vi "niFpgaPID_PIDCore.vi"(0 "setpoint":sgl, 1 "reset? (F)":bool, 3 "channel (0)":u8, 5 "process variable":sgl, 7 "manual control":T2, 12 "gains":T5 {"filter coefficient" min=0 max=1; "proportional gain" step=0.125}, 13 "output range":T4={"output high (Inf)"=inf, "output low (-Inf)"=-inf}, 14 "setpoint weighting":T3={"proportional weighting (1)"=1.0, "derivative weighting (0)"=0.0} {"derivative weighting (0)" min=0 max=1; "proportional weighting (1)" min=0 max=1}) -> (4 "output":sgl, 6 "error":sgl, 8 "actions":T1)   [LabVIEW 2017]
uses:
  <vilib>/rvi/Analysis/control/PID/Typedef/niFpgaPID_PIDGains.ctl
  <vilib>/rvi/Analysis/control/PID/Typedef/niFpgaPID_OutputRange.ctl
  <vilib>/rvi/Analysis/control/PID/Typedef/niFpgaPID_SetpointWeightings.ctl
  <vilib>/rvi/Analysis/control/PID/Typedef/niFpgaPID_ManualControl.ctl
  <vilib>/rvi/Analysis/control/PID/Typedef/niFpgaPID_PIDActions.ctl
  <vilib>/rvi/Analysis/control/PID/Typedef/niFpgaPID_PIDParameters.ctl
  <vilib>/rvi/Analysis/control/PID/Typedef/niFpgaPID_PIDErrors.ctl
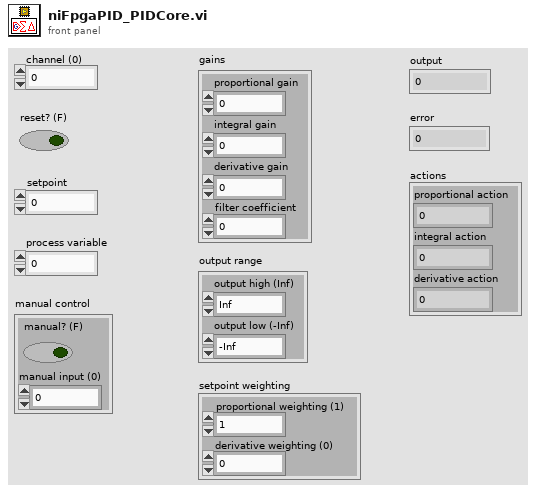
[diagram p1: front panel]
types:
  T1 = typedef "niFpgaPID_PIDActions.ctl" = cluster{"proportional action":sgl, "integral action":sgl, "derivative action":sgl}
  T2 = typedef "niFpgaPID_ManualControl.ctl" = cluster{"manual? (F)":bool, "manual input (0)":sgl}
  T3 = typedef "niFpgaPID_SetpointWeightings.ctl" = cluster{"proportional weighting (1)":sgl, "derivative weighting (0)":sgl}
  T4 = typedef "niFpgaPID_OutputRange.ctl" = cluster{"output high (Inf)":sgl, "output low (-Inf)":sgl}
  T5 = typedef "niFpgaPID_PIDGains.ctl" = cluster{"proportional gain":sgl, "integral gain":sgl, "derivative gain":sgl, "filter coefficient":sgl}
  T6 = typedef "niFpgaPID_PIDErrors.ctl" = cluster{"error":sgl, "error with beta":sgl, "error with gamma":sgl}
  T7 = typedef "niFpgaPID_PIDParameters.ctl" = cluster{"Kp":sgl, "Ki":sgl, "Kd":sgl, "manual?":bool, "beta":sgl}
  T8 = typedef "niFpgaPID_PIDState.ctl" = cluster{"uI(k-1)":sgl, "e(k-1)":sgl, "e(k-1) with gamma":sgl, "output (k-1)":sgl, "uD(k-1)":sgl}
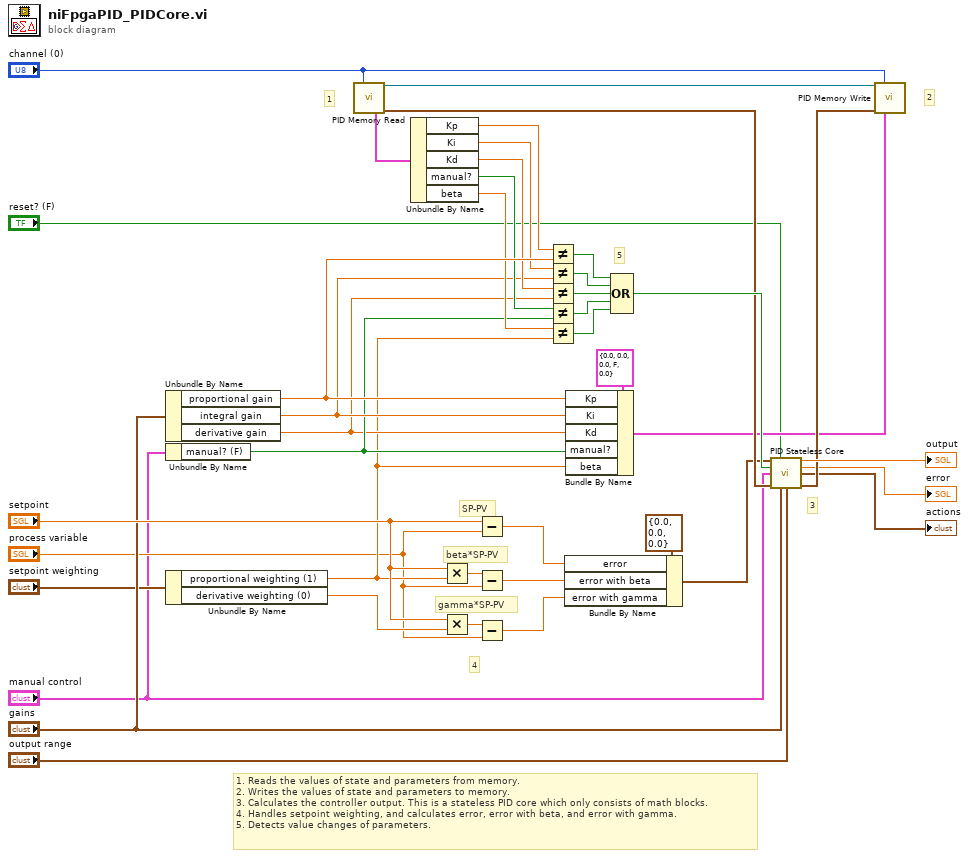
[diagram p0: block diagram]
diagram:
  # "SP-PV"
  # "beta*SP-PV"
  # "gamma*SP-PV"
  # "1. Reads the values of state and parameters from memory.\n2. Writes the values of state and parameters to memory.\n3. Calculates the controller output. This is a stateless PID core which only consists of math blocks.\n4. Handles setpoint weighting, and calculates error, error with beta, and error with gamma.\n5. Detects value changes of parameters."
  # "5"
  # "4"
  # "3"
  # "2"
  # "1"
  n1 = Unbundle By Name("gains") -> ("proportional gain"=w37:sgl, "integral gain"=w29:sgl, "derivative gain"=w27:sgl)
  n2 = Unbundle By Name("manual control") -> ("manual? (F)"=w28:bool)
  n3 = Unbundle By Name("setpoint weighting") -> ("proportional weighting (1)"=w16:sgl, "derivative weighting (0)"=w39:sgl)
  n4 = call "PID Memory Read"("channel (0)"="channel (0)") -> ("memory out"=w14:refnum<k21>, "parameters out"=w13:T7, "state out"=w35:T8)  [unwired: 12 in]
  n5 = Unbundle By Name(w13) -> ("Kp"=w34:sgl, "Ki"=w33:sgl, "Kd"=w32:sgl, "manual?"=w31:bool, "beta"=w30:sgl)
  n6 = Multiply(x="setpoint", y=w16) -> (x*y=w1:sgl)
  n7 = Multiply(x="setpoint", y=w39) -> (x*y=w2:sgl)
  n8 = Subtract(x="setpoint", y="process variable") -> (x-y=w5:sgl)
  n9 = Subtract(x=w1, y="process variable") -> (x-y=w10:sgl)
  n10 = Subtract(x=w2, y="process variable") -> (x-y=w9:sgl)
  n11 = Not Equal?(x=w34, y=w37) -> (x != y?=w26:bool)
  n12 = Not Equal?(x=w33, y=w29) -> (x != y?=w25:bool)
  n13 = Not Equal?(x=w32, y=w27) -> (x != y?=w24:bool)
  n14 = Not Equal?(x=w31, y=w28) -> (x != y?=w23:bool)
  n15 = Not Equal?(x=w30, y=w16) -> (x != y?=w22:bool)
  n16 = Bundle By Name(cluster=T6 {"error"=0.0, "error with beta"=0.0, "error with gamma"=0.0} ("errors"), "error"=w5, "error with beta"=w10, "error with gamma"=w9) -> (w8:T6)
  n17 = Bundle By Name(cluster=T7 {"Kp"=0.0, "Ki"=0.0, "Kd"=0.0, "manual?"=FALSE, "beta"=0.0} ("parameters"), "Kp"=w37, "Ki"=w29, "Kd"=w27, "manual?"=w28, "beta"=w16) -> (w12:T7)
  n18 = Compound Arithmetic op=OR(w26, w25, w24, w23, w22) -> (w38:bool)
  n19 = call "PID Stateless Core"("errors"=w8, "reset? (F)"="reset? (F)", "enable bumpless transfer? (F)"=w38, "manual control"="manual control", "state in"=w35, "gains"="gains", "output range"="output range") -> ("output"=→"output":sgl, "error"=→"error":sgl, "actions"=→"actions":T1, "state out"=w36:T8)  [unwired: 5 in]
  n20 = call "PID Memory Write"("memory in"=w14, "channel (0)"="channel (0)", "state in"=w36, "parameters in"=w12) -> ()  [unwired: 12 in]
